vi "WT300 Collect Raw Data.vi"(8 "error in (no error)":errorcluster, 11 "VISA Refnum in":refnum<visa-resource-name>) -> (0 "error out":errorcluster, 1 "Headers":string[](array[string]), 2 "Data":dbl[](array[numeric]), 3 "VISA resource name out":refnum<visa-resource-name>)   [LabVIEW 2018]
uses:
  <vilib>/Utility/error.llb/whitespace.ctl
  Public/Data/Read Measurement (Normal).vi
  Yokogawa WT300 Series.lvlib
panel:
  out "Array":bool[](array[boolean])
  out "All Headers Match":bool
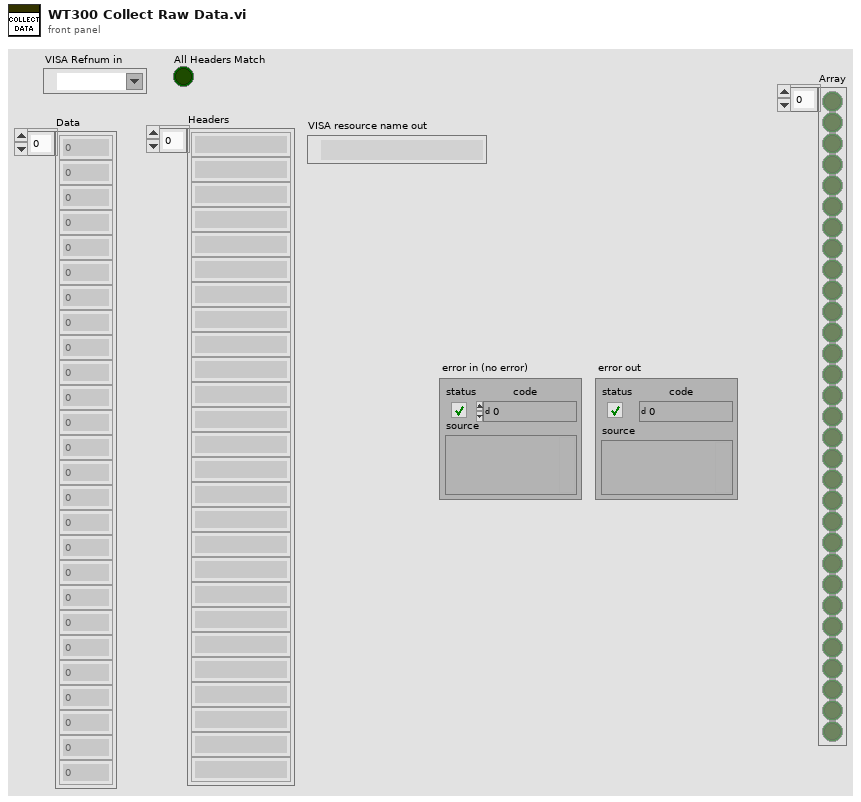
[diagram p1: front panel]
types:
  T1 = typedef "whitespace.ctl" = u16
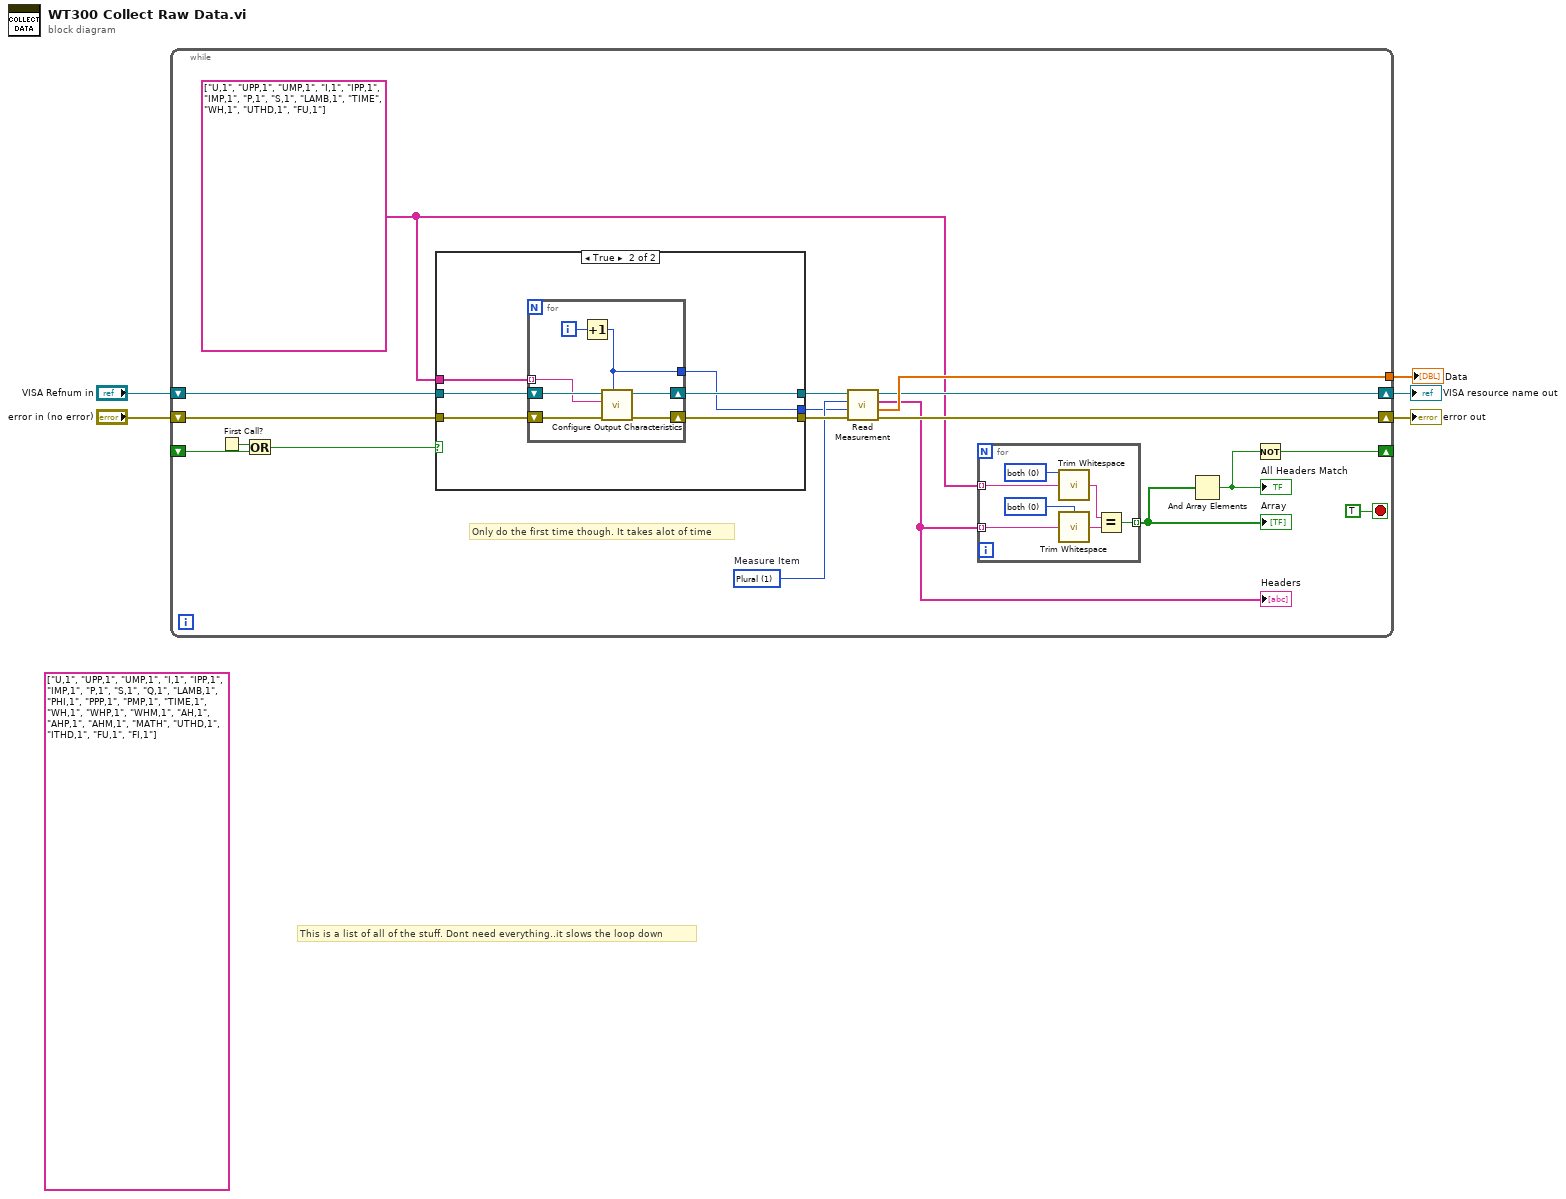
[diagram p0: block diagram]
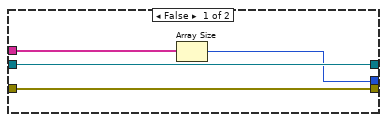
[diagram p2: hidden frame]
diagram:
  (unwired) string[] ["U,1", "UPP,1", "UMP,1", "I,1", "IPP,1", "IMP,1", "P,1", "S,1", "Q,1", "LAMB,1", "PHI,1", "PPP,1", "PMP,1", "TIME,1", "WH,1", "WHP,1", "WHM,1", "AH,1", "AHP,1", "AHM,1", "MATH", "UTHD,1", "ITHD,1", "FU,1", "FI,1"] ("appended array 2")
  # "This is a list of all of the stuff. Dont need everything..it slows the loop down"
  n1 = while {
    tunnel: [w19] -> w4
    shift-right: [w17] -> w3
    shift-left: "VISA Refnum in" -> [w23]
    shift-right: [w16] -> w2
    shift-left: "error in (no error)" -> [w15]
    shift-right: [w9] -> _
    shift-left: _ -> [w7]
    stop <- TRUE stop-if-true
    w12 = string[] ["U,1", "UPP,1", "UMP,1", "I,1", "IPP,1", "IMP,1", "P,1", "S,1", "LAMB,1", "TIME", "WH,1", "UTHD,1", "FU,1"] ("appended array 2")
    w20 = 1 items=["One", "Plural"]  # Measure Item
    # "Only do the first time though. It takes alot of time"
    n2 = First Call?() -> (First Call?: T/F=w8:bool)
    n3 = Or(x=w8, y=w7) -> (x .or. y?=w6:bool)
    n4 = case shown="True" w6 {
      tunnel: w12 -> [w32 w40]
      tunnel: w23 -> [w34 w39]
      tunnel: [w34 w38] -> w22
      tunnel: [w33 w37] -> w21
      tunnel: [w31 w36] -> w18
      tunnel: w15 -> [w33 w35]
      frame False {
        n5 = Array Size(array=w32) -> (size(s)=w31:i32)
      }
      frame True {
        n6 = for {
          shift-right: [w47] -> w38
          shift-left: w39 -> [w43]
          shift-right: [w46] -> w37
          shift-left: w35 -> [w44]
          tunnel: w40 -> [w42] mode=indexing
          tunnel: [w41] -> w36
          i -> [w45]
          n7 = Increment(x=w45) -> (x+1=w41:i32)
          n8 = call "Configure Output Characteristics.vi"("Item (1)"=w41, "error in (no error)"=w44, "Function (Empty)"=w42, "VISA resource name"=w43) -> ("error out"=w46:errorcluster, "VISA resource name out"=w47:refnum<visa-resource-name>)  [unwired: 6 in]
        }
      }
    }
    n9 = call-poly "Read Measurement.vi"("error in (no error)"=w21, "Number of Item (15)"=w18, "Measure Item (1: Plural)"=w20, "VISA resource name"=w22) -> ("error out"=w16:errorcluster, "Measurement"=w19:dbl[], "Function"=w13:string[], "VISA resource name out"=w17:refnum<visa-resource-name>)  [unwired: 4 in]
    "Headers" <- w13
    n10 = for {
      tunnel: w13 -> [w26] mode=indexing
      tunnel: w12 -> [w29] mode=indexing
      tunnel: [w30] -> w11 mode=indexing
      w24 = T1 0 items=["both", "start of string", "end of string"] ("location (both)")
      w25 = T1 0 items=["both", "start of string", "end of string"] ("location (both)")
      n11 = call <vilib>:"Trim Whitespace.vi"("string"=w29, "location (both)"=w25) -> ("trimmed string"=w28:string)
      n12 = call <vilib>:"Trim Whitespace.vi"("string"=w26, "location (both)"=w24) -> ("trimmed string"=w27:string)
      n13 = Equal?(x=w28, y=w27) -> (x = y?=w30:bool)
    }
    "Array" <- w11
    n14 = And Array Elements(Boolean array=w11) -> (logical AND=w10:bool)
    "All Headers Match" <- w10
    n15 = Not(x=w10) -> (.not. x?=w9:bool)
  }
  "Data" <- w4
  "VISA resource name out" <- w3
  "error out" <- w2
